vi "RelativePosition_KCubeDCServo.vi"(6 "set jog step size":dbl, 7 "lower limit":dbl, 8 "upper limit":dbl=25.0, 9 "Direction Control":enum16{"Backward", "Forward"}(ring), 10 "direction button":bool, 11 ".NET Refnum in":refnum<k24>) -> (0 "GetJogStepSize":dbl, 3 "error output":string)   [LabVIEW 2019]
doc: "set, get, and run relative position values for dc servo motor"
uses:
  D:/Victor Sun/optical trap control/Kinesis/ThorLabs.MotionControl.KCube.DCServoCLI.dll
  Kinesis/ThorLabs.MotionControl.KCube.DCServoCLI.dll
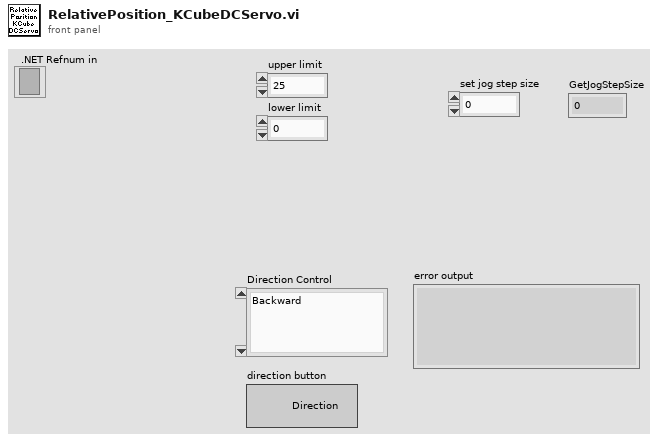
[diagram p1: front panel]
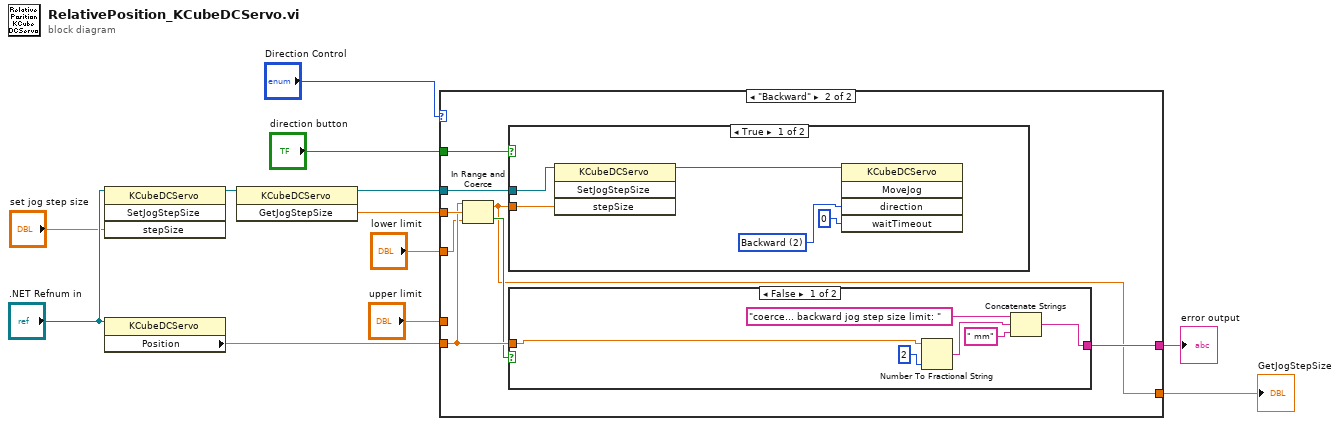
[diagram p0: block diagram]
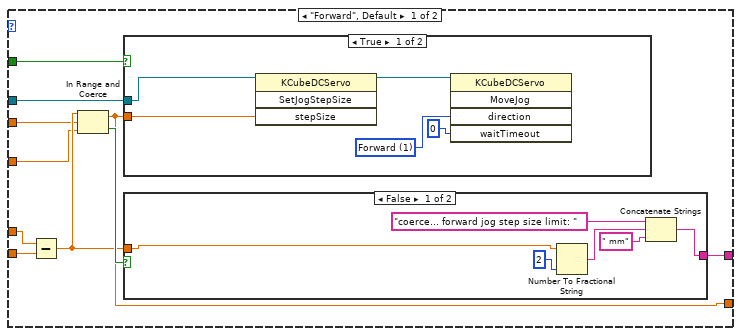
[diagram p2: hidden frame]
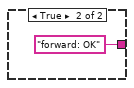
[diagram p3: hidden frame]
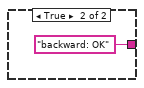
[diagram p5: hidden frame]
diagram:
  n1 = invoke class="KCubeDCServo" method="SetJogStepSize"(reference=".NET Refnum in", "stepSize"="set jog step size") -> (reference out=w3:refnum<k24>)  [unwired: 2 in, 3 out]
  n2 = property class="KCubeDCServo"(reference=".NET Refnum in") -> ("Position"=w9:dbl)  [unwired: 1 in, 2 out]
  n3 = invoke class="KCubeDCServo" method="GetJogStepSize"(reference=w3) -> (reference out=w11:refnum<k24>, "GetJogStepSize"=w8:dbl)  [unwired: 2 in, 1 out]
  n4 = case shown="\"Backward\"" "Direction Control" {
    tunnel: "direction button" -> [w20 w42]
    tunnel: w8 -> [w17 w41]
    tunnel: w9 -> [w18 w40]
    tunnel: [w16 w38] -> w10
    tunnel: w11 -> [w19 w37]
    tunnel: "lower limit" -> [w15 w36]
    tunnel: "upper limit" -> [w14 _]
    tunnel: [w13 w35] -> w1
    frame "Forward", Default {
      n5 = Subtract(x=w14, y=w18) -> (x-y=w21:dbl)
      n6 = In Range and Coerce(upper limit=w21, x=w17, lower limit=w15) -> (coerced(x)=w13:dbl, In Range?=w22:bool)
      n7 = case shown="True" w20 {
        tunnel: w19 -> [w31 _]
        tunnel: w13 -> [w30 _]
        frame True {
          w34 = 1 items=["Forward"=1, "Backward"=2] ("direction")
          n8 = invoke class="KCubeDCServo" method="SetJogStepSize"(reference=w31, "stepSize"=w30) -> (reference out=w32:refnum<k24>)  [unwired: 2 in, 3 out]
          n9 = invoke class="KCubeDCServo" method="MoveJog"(reference=w32, "direction"=w34, "waitTimeout"=0) -> ()  [unwired: 2 in, 5 out]
        }
        frame False {
        }
      }
      n10 = case shown="False" w22 {
        tunnel: w21 -> [w25 _]
        tunnel: [w23 "forward: OK"] -> w16
        frame False {
          n11 = Number To Fractional String(number=w25, precision (6)=i16 2) -> (F-format string=w28:string)  [unwired: 2 in]
          n12 = Concatenate Strings("coerce... forward jog step size limit: " ("string"), w28, " mm" ("string")) -> (w23:string)
        }
        frame True {
        }
      }
    }
    frame "Backward" {
      n13 = In Range and Coerce(upper limit=w40, x=w41, lower limit=w36) -> (coerced(x)=w35:dbl, In Range?=w39:bool)
      n14 = case shown="True" w42 {
        tunnel: w37 -> [w51 _]
        tunnel: w35 -> [w52 _]
        frame True {
          w54 = 2 items=["Forward"=1, "Backward"=2] ("direction")
          n15 = invoke class="KCubeDCServo" method="SetJogStepSize"(reference=w51, "stepSize"=w52) -> (reference out=w50:refnum<k24>)  [unwired: 2 in, 3 out]
          n16 = invoke class="KCubeDCServo" method="MoveJog"(reference=w50, "direction"=w54, "waitTimeout"=0) -> ()  [unwired: 2 in, 5 out]
        }
        frame False {
        }
      }
      n17 = case shown="False" w39 {
        tunnel: w40 -> [w44 _]
        tunnel: [w43 "backward: OK"] -> w38
        frame False {
          n18 = Number To Fractional String(number=w44, precision (6)=i16 2) -> (F-format string=w46:string)  [unwired: 2 in]
          n19 = Concatenate Strings("coerce... backward jog step size limit: " ("string"), w46, " mm" ("string")) -> (w43:string)
        }
        frame True {
        }
      }
    }
  }
  "error output" <- w10
  "GetJogStepSize" <- w1
